vi "AddOverlay.vi"(4 "Group":string="Points", 8 "error in (no error)":errorcluster, 10 "MarkersArray":T1, 11 "Refnum in":T3) -> (0 "error out":errorcluster, 3 "Refnum out":T3)   [LabVIEW 2017, in "ImageAcquisitionLibrary.lvlib"]
uses:
  ImageAcquisitionLibrary.lvlib
  <vilib>/vision/Image Controls.llb/IMAQ Image.ctl
  MarkersArray.ctl
  Marker.ctl
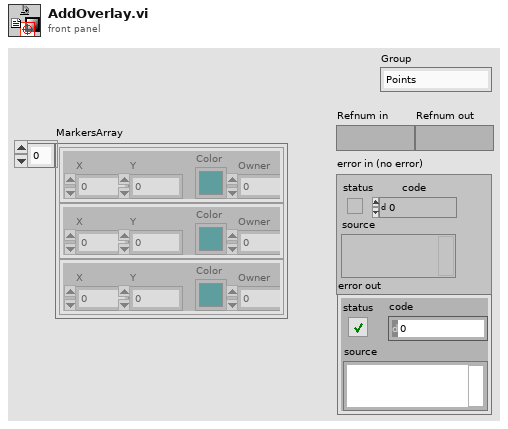
[diagram p1: front panel]
types:
  T1 = typedef "ImageAcquisitionLibrary.lvlib/MarkersArray.ctl" = T2[]
  T2 = typedef "ImageAcquisitionLibrary.lvlib/Marker.ctl" = cluster{"X":dbl, "Color":u32, "Y ":dbl, "Owner":u8}
  T3 = typedef "IMAQ Image.ctl" = refnum<image>
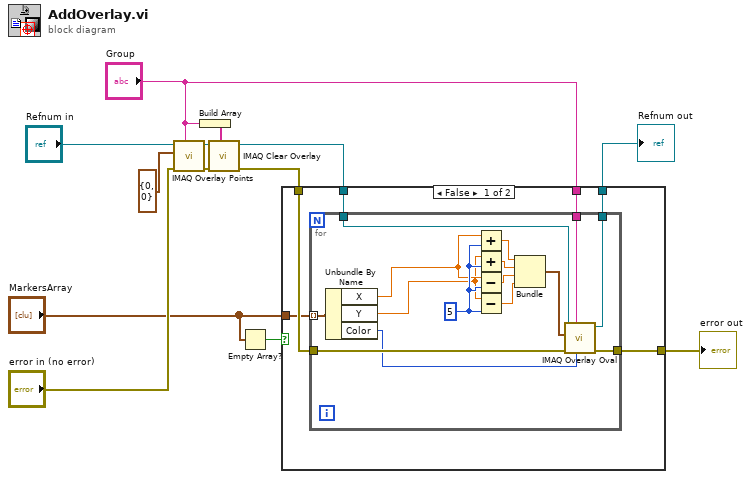
[diagram p0: block diagram]
diagram:
  n1 = call "IMAQ Overlay Points"("Group"="Group", "error in (no error)"="error in (no error)", "Point"=cluster{"X":i32, "Y":i32} {"X"=0, "Y"=0}, "Image"="Refnum in") -> ("error out"=w7:errorcluster, "Image Out"=w12:T3)  [unwired: 6 in]
  n2 = Build Array("Group") -> (w8:string[])
  n3 = call "IMAQ Clear Overlay"("Groups"=w8, "error in (no error)"=w7, "Image"=w12) -> ("error out"=w1:errorcluster, "Image Out"=w10:T3)  [unwired: 7 in]
  n4 = Empty Array?(array="MarkersArray") -> (empty?=w5:bool)
  n5 = case shown="False" w5 {
    tunnel: [w19 w36] -> w13
    tunnel: w10 -> [w18 w36]
    tunnel: "Group" -> [w17 _]
    tunnel: w1 -> [w16 w35]
    tunnel: [w15 w35] -> w6
    tunnel: "MarkersArray" -> [w14 _]
    frame False {
      n6 = for {
        tunnel: w14 -> [w23] mode=indexing
        tunnel: w18 -> [w28]
        tunnel: [w27] -> w19
        tunnel: w17 -> [w26]
        tunnel: w16 -> [w25]
        tunnel: [w24] -> w15
        w29 = 5 ("y")
        n7 = Unbundle By Name(w23) -> ("X"=w22:dbl, "Y"=w21:dbl, "Color"=w20:u32)
        n8 = Add(x=w22, y=w29) -> (x+y=w34:dbl)
        n9 = Add(x=w21, y=w29) -> (x+y=w33:dbl)
        n10 = Subtract(x=w22, y=w29) -> (x-y=w31:dbl)
        n11 = Subtract(x=w21, y=w29) -> (x-y=w32:dbl)
        n12 = Bundle(w34, w33, w31, w32) -> (w30:cluster{dbl, dbl, dbl, dbl})  [unwired: 1 in]
        n13 = call "IMAQ Overlay Oval"("Color"=w20, "Group"=w26, "error in (no error)"=w25, "Bounding Rectangle"=w30, "Image"=w28) -> ("error out"=w24:errorcluster, "Image Out"=w27:T3)  [unwired: 5 in]
      }
    }
    frame True {
    }
  }
  "Refnum out" <- w13
  "error out" <- w6
